vi "analyseData.vi"(8 "error in (no error)":errorcluster, 10 "HGF_VariantDataObject in":refnum<class "HGF_VariantDataObject.lvclass">, 11 "HGF_DataAnalysis in":refnum<class "HGF_DataAnalysis.lvclass">) -> (0 "error out":errorcluster, 2 "HGF_VariantDataObject out":refnum<class "HGF_VariantDataObject.lvclass">, 3 "HGF_DataAnalysis out":refnum<class "HGF_DataAnalysis.lvclass">)   [LabVIEW 2012, in "HGF_DataAnalyzer.lvlib" / "HGF_DataAnalysis.lvclass"]
doc: "Analyse data contained in HGF_DataVariantObject by using the HGF_DataAnalysator objects and optionally compining their results for a summaray result.\n\nThis is a dynamic dispatch VI to be overwritten by child classes."
uses:
  HGF_DataAnalysis.lvclass
  HGF_LVC/HGF_BaseClasses/HGF_VariantDataObject/HGF_VariantDataObject.lvclass
  HGF_LVC/HGF_BaseClasses/HGF_Composite/HGF_Composite.lvclass
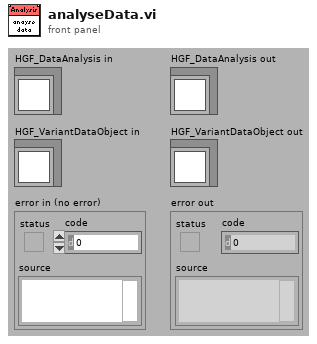
[diagram p1: front panel]
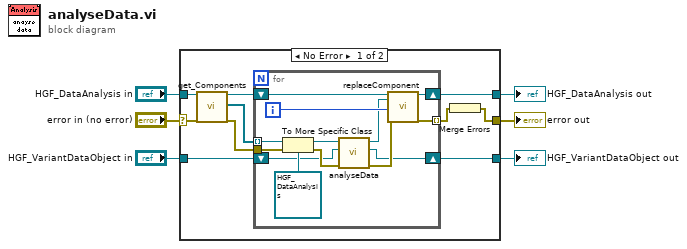
[diagram p0: block diagram]
diagram:
  n1 = case shown="No Error" "error in (no error)" {
    selector: "error in (no error)" -> [w15 w32]
    tunnel: [w10 w32] -> w5
    tunnel: [w8 w31] -> w3
    tunnel: "HGF_DataAnalysis in" -> [w16 w31]
    tunnel: "HGF_VariantDataObject in" -> [w12 w30]
    tunnel: [w7 w30] -> w1
    frame No Error {
      n2 = call "get_Components.vi"("HGF_Composite"=w16, "error in (no error)"=w15) -> ("dup HGF_Composite"=w9:refnum<class "HGF_DataAnalysis.lvclass">, "Components"=w14:refnum<class "HGF_Component.lvclass">[], "error out"=w13:errorcluster)  [unwired: 15 in]
      n3 = for {
        tunnel: w14 -> [w29] mode=indexing
        tunnel: w13 -> [w27]
        tunnel: [w18] -> w11 mode=indexing
        shift-right: [w22] -> w8
        shift-left: w9 -> [w23]
        shift-right: [w17] -> w7
        shift-left: w12 -> [w24]
        i -> [w21]
        n4 = To More Specific Class(target class=refnum<class "HGF_DataAnalysis.lvclass"> refnum ("HGF_DataAnalyzer.lvlib:HGF_DataAnalysis.lvclass"), reference=w29, error in=w27) -> (specific class reference=w28:refnum<class "HGF_DataAnalysis.lvclass">, error out=w26:errorcluster)
        n5 = call-dynamic "analyseData.vi"("error in (no error)"=w26, "HGF_VariantDataObject in"=w24, "HGF_DataAnalysis in"=w28) -> ("error out"=w19:errorcluster, "HGF_VariantDataObject out"=w17:refnum<class "HGF_VariantDataObject.lvclass">, "HGF_DataAnalysis out"=w20:refnum<class "HGF_DataAnalysis.lvclass">)  [unwired: 6 in]
        n6 = call "replaceComponent.vi"("HGF_Composite"=w23, "HGF_Component"=w20, "objectIndex"=w21, "error in (no error)"=w19) -> ("dup HGF_Composite"=w22:refnum<class "HGF_DataAnalysis.lvclass">, "error out"=w18:errorcluster)  [unwired: 14 in]
      }
      n7 = Merge Errors(w11) -> (w10:errorcluster)
    }
    frame Error {
    }
  }
  "error out" <- w5
  "HGF_DataAnalysis out" <- w3
  "HGF_VariantDataObject out" <- w1
